vi "Load Icon.vi"(8 "error in (no error)":errorcluster, 9 "Icon path True":path, 10 "Icon path False":path, 11 "Control in":refnum<class "Control.lvclass">) -> (0 "error out":errorcluster, 3 "Control out":refnum<class "Control.lvclass">)   [LabVIEW 2013, in "uitools_Control.lvlib" / "Control.lvclass"]
uses:
  Control.lvclass
  Control.lvclass/Control.ctl
  <userlib>/_OpenG.lib/file/file.llb/Strip Path - Traditional__ogtk.vi
  <userlib>/_OpenG.lib/file/file.llb/Strip Path Extension - String__ogtk.vi
  <userlib>/BitMan/BitMap class/BitMap.lvclass
  <userlib>/BitMan/Built-in Filters class/Built-in Filters.lvclass
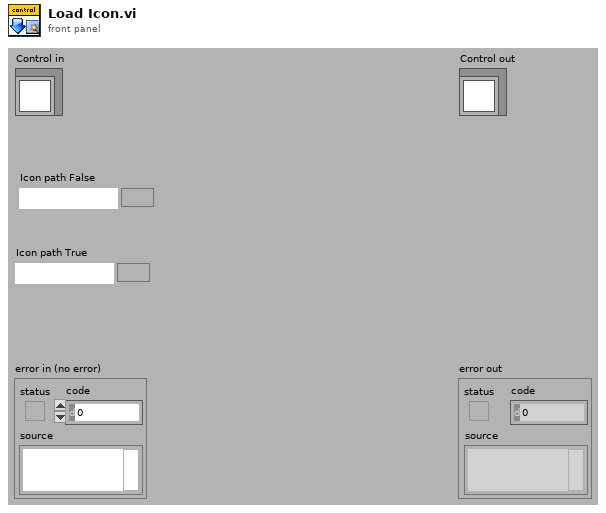
[diagram p1: front panel]
types:
  T1 = typedef "imagedata.ctl" = cluster{"image type":i32, "image depth":i32, "image":u8[], "mask":u8[], "colors":u32[], "Rectangle":cluster{"left":i16, "top":i16, "right":i16, "bottom":i16}}
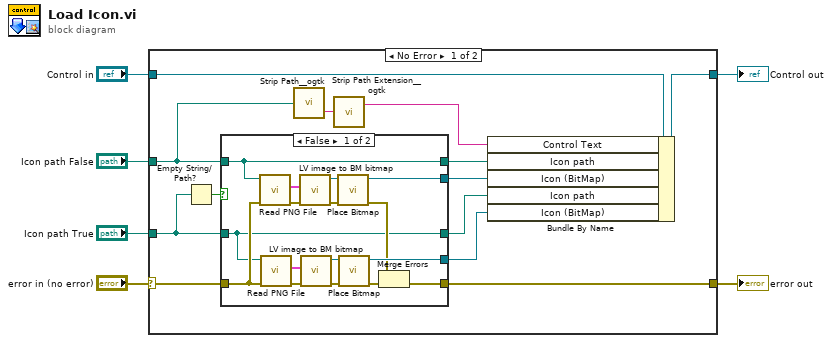
[diagram p0: block diagram]
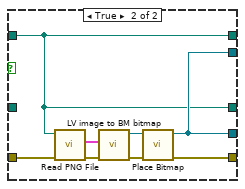
[diagram p2: hidden frame]
diagram:
  n1 = case shown="No Error" "error in (no error)" {
    selector: "error in (no error)" -> [w11 w45]
    tunnel: [w14 w45] -> w5
    tunnel: [w19 w44] -> w4
    tunnel: "Control in" -> [w16 w44]
    tunnel: "Icon path False" -> [w9 _]
    tunnel: "Icon path True" -> [w12 _]
    frame No Error {
      n2 = Empty String/Path?(string/path=w12) -> (empty?=w13:bool)
      n3 = case shown="False" w13 {
        tunnel: w12 -> [w21 _]
        tunnel: [w31 w39] -> w15
        tunnel: [w22 w38] -> w14
        tunnel: [w28 w39] -> w7
        tunnel: w9 -> [w20 w36]
        tunnel: w11 -> [w25 w37]
        tunnel: [w21 w36] -> w10
        tunnel: [w20 w36] -> w8
        frame False {
          n4 = call <vilib>:"Read PNG File.vi"("error in (no error)"=w25, "path to PNG file"=w20) -> ("error out"=w27:errorcluster, "image data"=w29:T1)  [unwired: 8 out]
          n5 = call <vilib>:"Read PNG File.vi"("error in (no error)"=w25, "path to PNG file"=w21) -> ("error out"=w34:errorcluster, "image data"=w35:T1)  [unwired: 8 out]
          n6 = call <userlib>:"LV image to BM bitmap.vi"("error in (no error)"=w27, "LV image data"=w29) -> ("error out"=w26:errorcluster, "BitMap out"=w30:refnum<class "BitMap.lvclass">)  [unwired: 2 in, 6 out]
          n7 = call <userlib>:"LV image to BM bitmap.vi"("error in (no error)"=w34, "LV image data"=w35) -> ("error out"=w33:errorcluster, "BitMap out"=w32:refnum<class "BitMap.lvclass">)  [unwired: 2 in, 6 out]
          n8 = call <userlib>:"Place Bitmap.vi"("error in (no error)"=w26, "Bitmap in (optional)"=w30) -> ("error out"=w24:errorcluster, "Bitmap out"=w28:refnum<class "BitMap.lvclass">)  [unwired: 4 in, 4 out]
          n9 = call <userlib>:"Place Bitmap.vi"("error in (no error)"=w33, "Bitmap in (optional)"=w32) -> ("error out"=w23:errorcluster, "Bitmap out"=w31:refnum<class "BitMap.lvclass">)  [unwired: 4 in, 4 out]
          n10 = Merge Errors(w24, w23) -> (w22:errorcluster)
        }
        frame True {
          n11 = call <vilib>:"Read PNG File.vi"("error in (no error)"=w37, "path to PNG file"=w36) -> ("error out"=w42:errorcluster, "image data"=w43:T1)  [unwired: 8 out]
          n12 = call <userlib>:"LV image to BM bitmap.vi"("error in (no error)"=w42, "LV image data"=w43) -> ("error out"=w41:errorcluster, "BitMap out"=w40:refnum<class "BitMap.lvclass">)  [unwired: 2 in, 6 out]
          n13 = call <userlib>:"Place Bitmap.vi"("error in (no error)"=w41, "Bitmap in (optional)"=w40) -> ("error out"=w38:errorcluster, "Bitmap out"=w39:refnum<class "BitMap.lvclass">)  [unwired: 4 in, 4 out]
        }
      }
      n14 = call-poly <userlib>:"Strip Path__ogtk.vi"("path"=w9) -> ("name"=w18:string)  [unwired: 1 out]
      n15 = call-poly <userlib>:"Strip Path Extension__ogtk.vi"("path"=w18) -> ("root"=w17:string)  [unwired: 1 out]
      n16 = Bundle By Name(cluster=w16, "Control Text"=w17, "Icon path"=w8, "Icon (BitMap)"=w7, "Icon path"=w10, "Icon (BitMap)"=w15) -> (w19:refnum<class "Control.lvclass">)
    }
    frame Error {
    }
  }
  "error out" <- w5
  "Control out" <- w4
